vi "Perform Action.vi"(7 "Instrument":refnum<class "Instrument.lvclass">, 8 "error in":errorcluster, 10 "Input":variant, 11 "object in":refnum<class "Perform Action on N Const Channels Strategy.lvclass">) -> (0 "error out":errorcluster, 2 "Output":variant, 3 "object out":refnum<class "Perform Action on N Const Channels Strategy.lvclass">)   [LabVIEW 2024, in "HAL.lvlib" / "Perform Action on N Const Channels Strategy.lvclass"]
uses:
  Perform Action on N Const Channels Strategy.lvclass
  Perform Action on N Const Channels Strategy.lvclass/Perform Action on N Const Channels Strategy.ctl
  Instrument/Instrument.lvclass
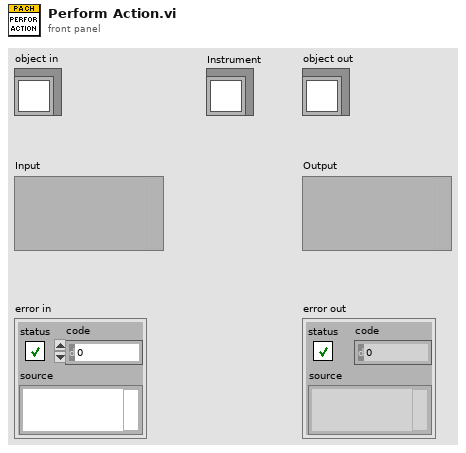
[diagram p1: front panel]
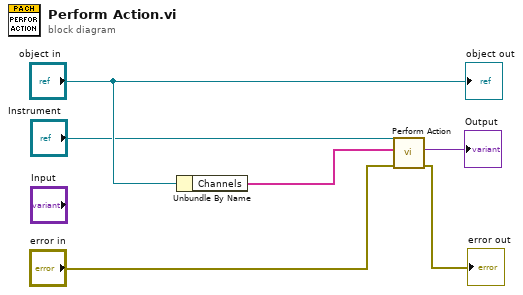
[diagram p0: block diagram]
diagram:
  n1 = Unbundle By Name("object in") -> ("Channels"=w5:string[])
  n2 = call "Perform Action.vi"("Error In"="error in", "Input"=w5, "reference in"="Instrument") -> ("Error Out"=→"error out":errorcluster, "Output"=→"Output":variant)  [unwired: 6 in, 1 out]
  "object out" <- "object in"
